vi "Trimmed data queue.vi"(4 "timeout in ms (-1)":i32=10, 6 "max queue size (-1, unlimited)":i32, 7 "Action":T1=enum."Enqueue", 8 "error in (no error)":errorcluster, 11 "data in":sgl[](array[numeric])) -> (0 "error out":errorcluster, 1 "Empty?":bool, 2 "# elements in queue":i32, 3 "data out":sgl[](array[numeric]))   [LabVIEW 2018]
uses:
  Controls/Queue Manager Actions.ctl
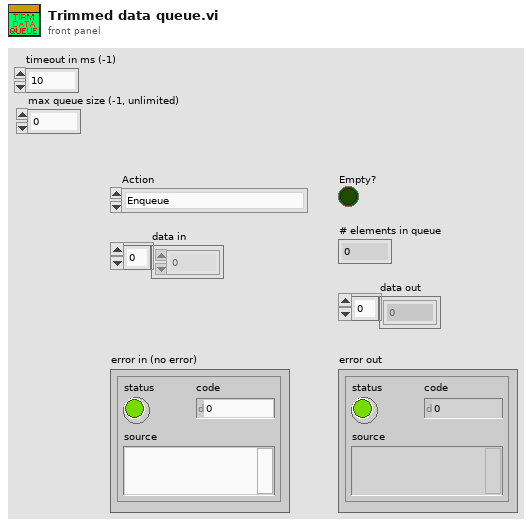
[diagram p1: front panel]
types:
  T1 = typedef "Queue Manager Actions.ctl" = enum16{"Init", "Enqueue", "Enqueue All", "Preview Queue", "Dequeue", "Get Status", "Flush Queue", "Flush All Queues", "Release All Queues", "Release Queue", "Enqueue at Opposite End"}
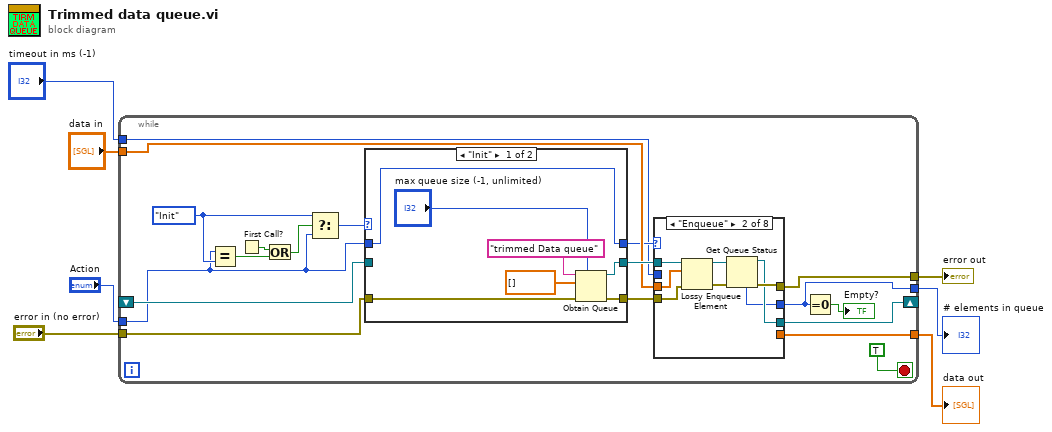
[diagram p0: block diagram]
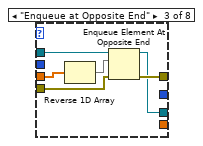
[diagram p3: hidden frame]
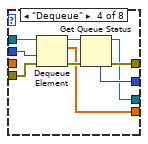
[diagram p4: hidden frame]
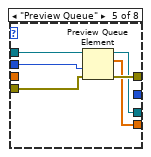
[diagram p5: hidden frame]
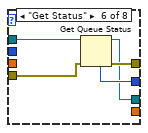
[diagram p6: hidden frame]
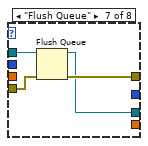
[diagram p7: hidden frame]
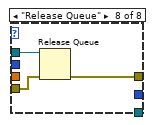
[diagram p8: hidden frame]
diagram:
  n1 = while {
    tunnel: "Action" -> [w9]
    tunnel: "error in (no error)" -> [w14]
    shift-right: [w16] -> _
    shift-left: _ -> [w15]
    tunnel: "data in" -> [w12]
    tunnel: "timeout in ms (-1)" -> [w8]
    tunnel: [w19] -> w3
    tunnel: [w18] -> w2
    tunnel: [w11] -> w1
    stop <- TRUE stop-if-true
    w21 = Queue_Manager_Actions."Init"
    n2 = Equal?(x=w9, y=w21) -> (x = y?=w23:bool)
    n3 = First Call?() -> (First Call?: T/F=w24:bool)
    n4 = Or(x=w24, y=w23) -> (x .or. y?=w22:bool)
    n5 = Select(t=w21, s=w22, f=w9) -> (s? t:f=w20:T1)
    n6 = case shown="\"Init\"" w20 {
      tunnel: [w76 w79] -> w17
      tunnel: [w75 w78] -> w13
      tunnel: w15 -> [_ w79]
      tunnel: w14 -> [w73 w78]
      tunnel: [w71 w77] -> w10
      tunnel: w9 -> [w71 w77]
      frame "Init" {
        n7 = Obtain Queue(max queue size (-1, unlimited)="max queue size (-1, unlimited)", name (unnamed)="trimmed Data queue", element data type=sgl[] [], error in (no error)=w73) -> (queue out=w76:refnum<queue>, error out=w75:errorcluster)  [unwired: 1 in, 1 out]
      }
      frame Default {
      }
    }
    n8 = case shown="\"Enqueue\"" w10 {
      tunnel: [w27 w31 w42 w50 w57 w62 w66 w69] -> w19
      tunnel: [_ _ _ w47 w56 _ _ _] -> w18
      tunnel: [_ w29 _ w48 _ w61 _ _] -> w11
      tunnel: w17 -> [w28 w36 w39 w46 w54 w60 w65 w68]
      tunnel: [w28 w30 w40 w44 w53 w58 w63 _] -> w16
      tunnel: w13 -> [w27 w35 w38 w45 w55 w59 w64 w67]
      tunnel: w12 -> [_ w34 w37 _ _ _ _ _]
      tunnel: w8 -> [_ _ _ w43 w52 _ _ _]
      frame "Init", Default {
      }
      frame "Enqueue" {
        n9 = Lossy Enqueue Element(queue=w36, element=w34, error in (no error)=w35) -> (queue out=w33:refnum<queue>, error out=w32:errorcluster)  [unwired: 2 out]
        n10 = Get Queue Status(queue=w33, error in (no error)=w32) -> (queue out=w30:refnum<queue>, error out=w31:errorcluster, # elements in queue=w29:i32)  [unwired: 1 in, 5 out]
      }
      frame "Enqueue at Opposite End" {
        n11 = Reverse 1D Array(array=w37) -> (reversed array=w41:sgl[])
        n12 = Enqueue Element At Opposite End(queue=w39, element=w41, error in (no error)=w38) -> (queue out=w40:refnum<queue>, error out=w42:errorcluster)  [unwired: 1 in, 1 out]
      }
      frame "Dequeue" {
        n13 = Dequeue Element(queue=w46, timeout in ms (-1)=w43, error in (no error)=w45) -> (queue out=w49:refnum<queue>, element=w47:sgl[], error out=w51:errorcluster)  [unwired: 1 out]
        n14 = Get Queue Status(queue=w49, error in (no error)=w51) -> (queue out=w44:refnum<queue>, error out=w50:errorcluster, # elements in queue=w48:i32)  [unwired: 1 in, 5 out]
      }
      frame "Preview Queue" {
        n15 = Preview Queue Element(queue=w54, timeout in ms (-1)=w52, error in (no error)=w55) -> (queue out=w53:refnum<queue>, element=w56:sgl[], error out=w57:errorcluster)  [unwired: 1 out]
      }
      frame "Get Status" {
        n16 = Get Queue Status(queue=w60, error in (no error)=w59) -> (queue out=w58:refnum<queue>, error out=w62:errorcluster, # elements in queue=w61:i32)  [unwired: 1 in, 5 out]
      }
      frame "Flush Queue" {
        n17 = Flush Queue(queue=w65, error in (no error)=w64) -> (queue out=w63:refnum<queue>, error out=w66:errorcluster)  [unwired: 1 out]
      }
      frame "Release Queue" {
        n18 = Release Queue(queue=w68, error in (no error)=w67) -> (error out=w69:errorcluster)  [unwired: 1 in, 2 out]
      }
    }
    n19 = Equal To 0?(x=w11) -> (x = 0?=→"Empty?":bool)
  }
  "error out" <- w3
  "data out" <- w2
  "# elements in queue" <- w1
